vi "encode_camera_frames.vi"(8 "error in":errorcluster, 10 "Re-do":bool, 11 "Experiment Folder In":string) -> (0 "Error Out":errorcluster)   [LabVIEW 2019]
panel:
  out "Zip Image Index":i32
  out "Image Count":i32
  out "FFMPEG output":string
  out "FFMPEG command":string
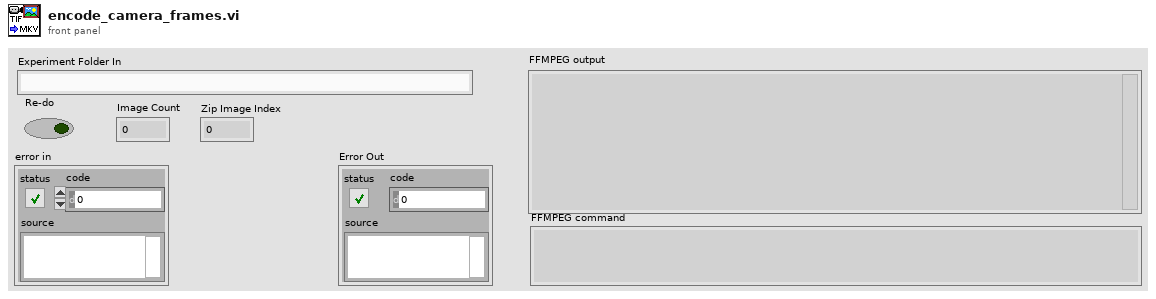
[diagram p1: front panel]
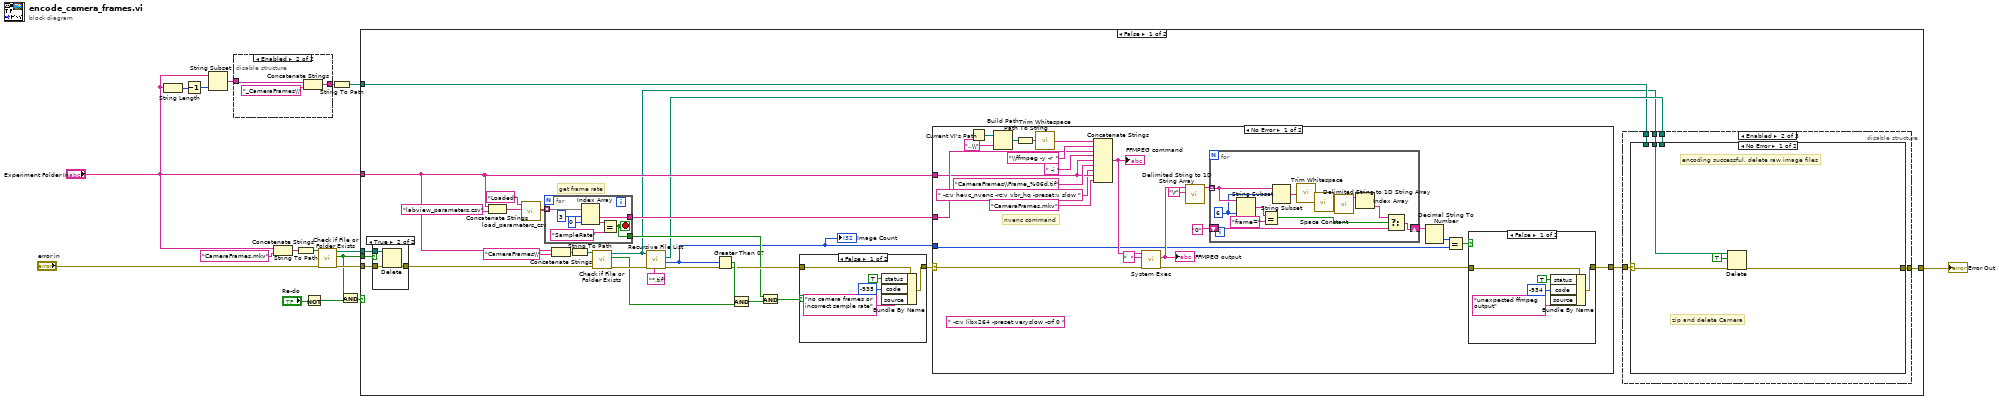
[diagram p0: block diagram]
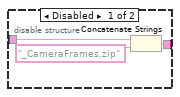
[diagram p2: hidden frame]
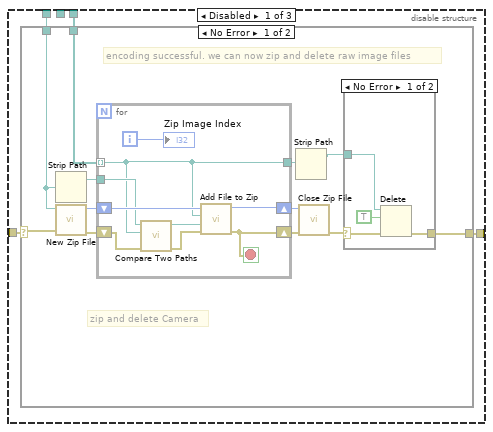
[diagram p3: hidden frame]
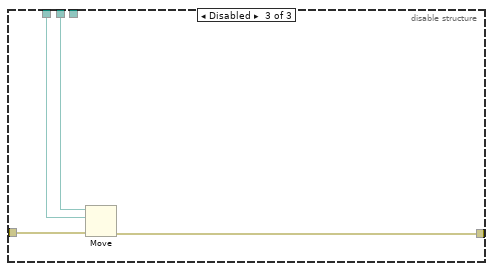
[diagram p7: hidden frame]
diagram:
  n1 = String Length(string="Experiment Folder In") -> (length=w5:i32)
  n2 = Decrement(x=w5) -> (x-1=w4:i32)
  n3 = String Subset(string="Experiment Folder In", length (rest)=w4) -> (substring=w3:string)  [unwired: 1 in]
  n4 = disable-structure shown="Enabled" {
    disable-tunnel: w3 -> [w19 w22]
    disable-tunnel: [w18 w21] -> w2
    frame Disabled {
      n5 = Concatenate Strings(w19, "_CameraFrames.zip" ("string")) -> (w18:string)
    }
    frame Enabled {
      n6 = Concatenate Strings(w22, "_CameraFrames\\" ("string")) -> (w21:string)
    }
  }
  n7 = Concatenate Strings("Experiment Folder In", "CameraFrames.mkv" ("string")) -> (w15:string)
  n8 = String To Path(string=w15) -> (path=w17:path)
  n9 = Not(x="Re-do") -> (.not. x?=w10:bool)
  n10 = call <vilib>:"Check if File or Folder Exists.vi"("error in (no error)"="error in", "path"=w17) -> ("error out"=w12:errorcluster, "file or folder exists?"=w8:bool, "dup path"=w7:path)  [unwired: 7 in]
  n11 = String To Path(string=w2) -> (path=w1:path)
  n12 = And(x=w8, y=w10) -> (x .and. y?=w9:bool)
  n13 = case shown="False" w9 {
    tunnel: "Experiment Folder In" -> [w51 _]
    tunnel: [w28 w158] -> w13
    tunnel: w12 -> [w50 w158]
    tunnel: w8 -> [w49 _]
    tunnel: w7 -> [w48 _]
    tunnel: w1 -> [w25 _]
    frame False {
      # "get frame rate"
      n14 = case shown="True" w49 {
        tunnel: [w97 w100] -> w30
        tunnel: w50 -> [w97 w99]
        tunnel: w48 -> [_ w98]
        frame False {
        }
        frame True {
          n15 = Delete(path (use dialog)=w98, error in=w99) -> (error out=w100:errorcluster)  [unwired: 3 in, 2 out]
        }
      }
      n16 = Concatenate Strings(w51, "labview_parameters.csv" ("string")) -> (w35:string)
      n17 = call "load_parameters_csv.vi"("Parameter CSV Path"=w35, "Tags In"="Loaded") -> ("Loaded Params"=w34:string[][])  [unwired: 6 in, 3 out]
      n18 = for {
        tunnel: w34 -> [w107] mode=indexing
        tunnel: [w102] -> w46
        tunnel: [w101] -> w31
        stop <- w101 stop-if-true
        n19 = Index Array(array=w107, index #1=3 ("index"), index #2=0 ("index")) -> (element #1=w102:string, element #2=w105:string)
        n20 = Equal?(x=w105, y="SampleRate") -> (x = y?=w101:bool)
      }
      n21 = Concatenate Strings(w51, "CameraFrames\\" ("string")) -> (w44:string)
      n22 = String To Path(string=w44) -> (path=w43:path)
      n23 = call <vilib>:"Check if File or Folder Exists.vi"("error in (no error)"=w30, "path"=w43) -> ("error out"=w41:errorcluster, "file or folder exists?"=w39:bool, "dup path"=w24:path)  [unwired: 7 in]
      n24 = call <vilib>:"Recursive File List.vi"("pattern"="*.tif", "error in (no error)"=w41, "Folder Path"=w24) -> ("error out"=w38:errorcluster, "Number of Files"=w26:i32, "All Files in Dir"=w27:path[])  [unwired: 4 in, 2 out]
      "Image Count" <- w26
      n25 = Greater Than 0?(x=w26) -> (x > 0?=w40:bool)
      n26 = And(x=w40, y=w39) -> (x .and. y?=w33:bool)
      n27 = And(x=w31, y=w33) -> (x .and. y?=w32:bool)
      n28 = case shown="False" w32 {
        tunnel: w38 -> [w112 w113]
        tunnel: [w108 w113] -> w47
        frame False {
          n29 = Bundle By Name(cluster=w112, "status"=TRUE, "code"=-935, "source"="no camera frames or incorrect sample rate") -> (w108:errorcluster)
        }
        frame True {
        }
      }
      n30 = case shown="No Error" w47 {
        selector: w47 -> [w126 w157]
        tunnel: w46 -> [w132 _]
        tunnel: [w119 w157] -> w29
        tunnel: w51 -> [w129 _]
        tunnel: w26 -> [w121 _]
        frame No Error {
          (unwired) " -c:v libx264 -preset veryslow -crf 0 "
          # "nvenc command"
          n31 = Current VI's Path() -> (path=w136:path)
          n32 = Build Path(base path=w136, name or relative path="..\\") -> (appended path=w137:path)
          n33 = Path To String(path=w137) -> (string=w138:string)
          n34 = call <vilib>:"Trim Whitespace.vi"("string"=w138) -> ("trimmed string"=w135:string)  [unwired: 1 in]
          n35 = Concatenate Strings(w135, "\\ffmpeg -y -r  " ("string"), w132, " -i " ("string"), w129, "CameraFrames\\Frame_%06d.tif" ("string"), " -c:v hevc_nvenc -rc:v vbr_hq -preset:v slow " ("string"), w129, "CameraFrames.mkv" ("string")) -> (w125:string)
          "FFMPEG command" <- w125
          n36 = call <vilib>:"System Exec.vi"("error in (no error)"=w126, "standard input"="  ", "command line"=w125) -> ("error out"=w120:errorcluster, "standard error"=w124:string)  [unwired: 5 in, 2 out]
          "FFMPEG output" <- w124
          n37 = call <vilib>:"Delimited String to 1D String Array.vi"("delimiter"="\r", "delimited string"=w124) -> ("string array"=w116:string[])  [unwired: 9 in]
          n38 = for {
            tunnel: w116 -> [w144] mode=indexing
            shift-right: [w147] -> w114
            shift-left: "0" ("y") -> [w148]
            w143 = 6 ("length (rest)")
            n39 = String Subset(string=w144, length (rest)=w143) -> (substring=w145:string)  [unwired: 1 in]
            n40 = Equal?(x=w145, y="frame=") -> (x = y?=w149:bool)
            n41 = String Subset(string=w144, offset (0)=w143) -> (substring=w141:string)  [unwired: 1 in]
            n42 = call <vilib>:"Trim Whitespace.vi"("string"=w141) -> ("trimmed string"=w140:string)  [unwired: 1 in]
            n43 = call <vilib>:"Space Constant.vi"() -> ("String"=w146:string)
            n44 = call <vilib>:"Delimited String to 1D String Array.vi"("delimiter"=w146, "delimited string"=w140) -> ("string array"=w142:string[])  [unwired: 9 in]
            n45 = Index Array(array=w142) -> (element=w139:string)  [unwired: 1 in]
            n46 = Select(t=w139, s=w149, f=w148) -> (s? t:f=w147:string)
          }
          n47 = Decimal String To Number(string=w114) -> (number=w122:i32)  [unwired: 2 in, 1 out]
          n48 = Equal?(x=w122, y=w121) -> (x = y?=w118:bool)
          n49 = case shown="False" w118 {
            tunnel: w120 -> [w155 w156]
            tunnel: [w151 w156] -> w119
            frame False {
              n50 = Bundle By Name(cluster=w155, "status"=TRUE, "code"=-934, "source"="unexpected ffmpeg output") -> (w151:errorcluster)
            }
            frame True {
            }
          }
        }
        frame Error {
        }
      }
      n51 = disable-structure shown="Enabled" {
        disable-tunnel: w29 -> [w55 w87 w96]
        disable-tunnel: [w54 w86 w95] -> w28
        disable-tunnel: w27 -> [w53 w85 _]
        disable-tunnel: w25 -> [w52 w84 w94]
        disable-tunnel: w24 -> [_ w83 w93]
        frame Disabled {
          n52 = case shown="No Error" w55 {
            selector: w55 -> [w58 w82]
            tunnel: [w57 w82] -> w54
            tunnel: w53 -> [w65 _]
            tunnel: w52 -> [w56 _]
            frame No Error {
              # "zip and delete Camera"
              # "encoding successful. we can now zip and delete raw image files"
              n53 = Strip Path(path=w56) -> (stripped path=w62:path)  [unwired: 1 out]
              n54 = call <vilib>:"New Zip File.vi"("error in (no error)"=w58, "target"=w56) -> ("error out"=w64:errorcluster, "zip file out"=w63:i64)  [unwired: 3 in, 1 out]
              n55 = for {
                tunnel: w65 -> [w69] mode=indexing
                shift-right: [w75] -> w60
                shift-left: w63 -> [w76]
                shift-right: [w72] -> w61
                shift-left: w64 -> [w74]
                tunnel: w62 -> [w71]
                tunnel: [w69] -> w59
                i -> [w68]
                stop <- w72 stop-if-true
                n56 = call <vilib>:"Compare Two Paths.vi"("error in (no error)"=w74, "Path 2"=w69, "Path 1"=w71) -> ("error out"=w73:errorcluster, "Relative Path from 1 to 2"=w70:path)  [unwired: 5 in, 2 out]
                n57 = call <vilib>:"Add File to Zip.vi"("error in (no error)"=w73, "destination path in zip"=w70, "source file path"=w69, "zip file in"=w76) -> ("error out"=w72:errorcluster, "zip file out"=w75:i64)  [unwired: 6 in]
                "Zip Image Index" <- w68
              }
              n58 = Strip Path(path=w59) -> (stripped path=w66:path)  [unwired: 1 out]
              n59 = call <vilib>:"Close Zip File.vi"("error in (no error)"=w61, "zip file in"=w60) -> ("error out"=w67:errorcluster)  [unwired: 1 in, 4 out]
              n60 = case shown="No Error" w67 {
                selector: w67 -> [w79 w81]
                tunnel: [w78 w81] -> w57
                tunnel: w66 -> [w77 _]
                frame No Error {
                  n61 = Delete(path (use dialog)=w77, entire hierarchy (F)=TRUE, error in=w79) -> (error out=w78:errorcluster)  [unwired: 2 in, 2 out]
                }
                frame Error {
                }
              }
            }
            frame Error {
            }
          }
        }
        frame Enabled {
          n62 = case shown="No Error" w87 {
            selector: w87 -> [w89 w92]
            tunnel: [w91 w92] -> w86
            tunnel: w85 -> [_ _]
            tunnel: w84 -> [_ _]
            tunnel: w83 -> [w88 _]
            frame No Error {
              # "zip and delete Camera"
              # "encoding successful. delete raw image files"
              n63 = Delete(path (use dialog)=w88, entire hierarchy (F)=TRUE, error in=w89) -> (error out=w91:errorcluster)  [unwired: 2 in, 2 out]
            }
            frame Error {
            }
          }
        }
        frame Disabled {
          n64 = Move(source path=w93, error in=w96, 10:w94) -> (error out=w95:errorcluster)  [unwired: 2 in, 2 out]
        }
      }
    }
    frame True {
    }
  }
  "Error Out" <- w13
